vi "issueBootCommand.vi"(8 "error in (no error)":errorcluster, 11 "Boot in":refnum<class "Boot.lvclass">) -> (0 "error out":errorcluster, 3 "Boot out":refnum<class "Boot.lvclass">)   [LabVIEW 2016, in "Boot.lvclass"]
uses:
  Boot.lvclass
  DataTypes/General/ProcessCommandEvent.ctl
  Commands/Command/Command.lvclass
  Commands/BootCommand/BootCommand.lvclass
  D:/Code/ts_M1M3Support/Commands/Command/Command.lvclass
  Boot.lvclass/Boot.ctl
  UserEvents/UserEvents.lvclass/UserEvents.ctl
  UserEvents/UserEvents.lvclass
  DataTypes/General/M1M3SupportGeneral.lvlib
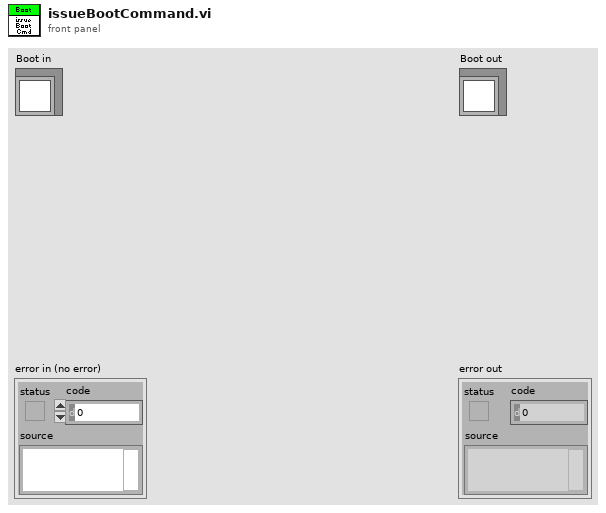
[diagram p1: front panel]
types:
  T1 = typedef "M1M3SupportGeneral.lvlib/ProcessCommandEvent.ctl" = cluster{"Command":refnum<class "Command.lvclass">}
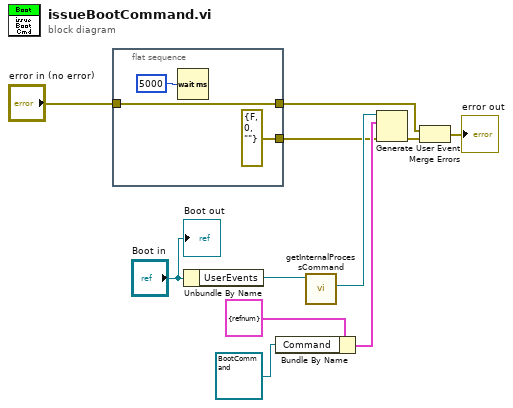
[diagram p0: block diagram]
diagram:
  n1 = flat-sequence {
    tunnel: [w13] -> w6
    tunnel: "error in (no error)" -> [w13]
    tunnel: [errorcluster {"status"=FALSE, "code"=0, "source"=""} ("error in (no error)")] -> w5
    frame #0 {
      n2 = Wait (ms)(milliseconds to wait=u32 5000) -> ()  [unwired: 1 out]
    }
  }
  n3 = Unbundle By Name("Boot in") -> ("UserEvents"=w1:refnum<class "UserEvents.lvclass">)
  n4 = Bundle By Name(cluster=T1 {"Command"=refnum} ("ProcessCommandEvent"), "Command"=refnum<class "BootCommand.lvclass"> refnum ("BootCommand.lvclass")) -> (w9:T1)
  n5 = call "getInternalProcessCommand.vi"("UserEvents in"=w1) -> ("InternalProcessCommand"=w8:refnum<user-event>)  [unwired: 9 in, 1 out]
  n6 = Generate User Event(user event=w8, event data cluster=w9, error in=w5) -> (error out=w4:errorcluster)  [unwired: 1 in, 1 out]
  n7 = Merge Errors(w6, w4) -> (→"error out":errorcluster)
  "Boot out" <- "Boot in"
